vi "Read Power Measurement Standard Deviation List Mode.vi"(8 "error in (no error)":errorcluster, 9 "Step Index (1)":i32=1, 10 "Instance (1)":i32=1, 11 "VISA resource name":refnum<visa-resource-name>) -> (0 "error out":errorcluster, 1 "Standard Deviation":dbl format="%^.3e", 2 "Reliability":i32, 3 "VISA resource name out":refnum<visa-resource-name>)   [LabVIEW 2015, in "Rohde&Schwarz CMXP GPRF.lvlib"]
doc: "Starts a new single shot measurement and returns the standard deviation of the selected <StepIndex> measurement result.\n\nAttribute:\n-\n\nRemote-control command:\nREAD:GPRF:MEAS<i>:POWer:LIST:SDEViation?"
uses:
  <instrlib>/Rohde&Schwarz CMXP GPRF/Rohde&Schwarz CMXP GPRF.lvlib
  <instrlib>/Rohde&Schwarz CMXP GPRF/Private/rsidr_core.llb/rsidr_core.lvlib
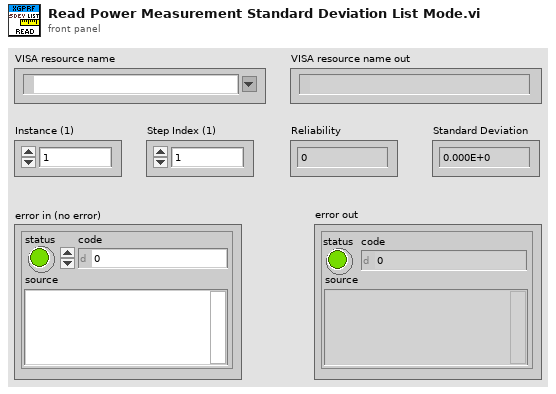
[diagram p1: front panel]
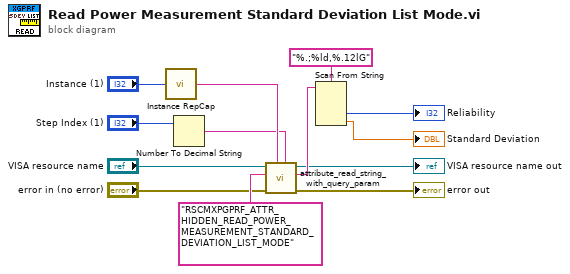
[diagram p0: block diagram]
diagram:
  n1 = call <instrlib>:"Instance RepCap.vi"("instance  in"="Instance (1)") -> ("instance out"=w13:string)
  n2 = Number To Decimal String(number="Step Index (1)") -> (decimal integer string=w11:string)  [unwired: 1 in]
  n3 = call <instrlib>:"attribute_read_string_with_query_param.vi"("Query Parameter (None)"=w11, "Repeated Capability (\"\")"=w13, "error in"="error in (no error)", "Attribute ID"="RSCMXPGPRF_ATTR_HIDDEN_READ_POWER_MEASUREMENT_STANDARD_DEVIATION_LIST_MODE", "VISA resource name"="VISA resource name") -> ("error out"=→"error out":errorcluster, "String out"=w9:string, "VISA resource name out"=→"VISA resource name out":refnum<visa-resource-name>)  [unwired: 4 in]
  n4 = Scan From String(format string="%.;%ld,%.12lG", input string=w9) -> (output 1=→"Reliability":i32, output 2=→"Standard Deviation":dbl)  [unwired: 4 in, 3 out]
